vi "Set Position For Align Or Distribute.vi"(8 "Error In":errorcluster, 9 "Position":i32, 10 "Vertical? (F: Horizontal)":bool, 11 "Splitter in":refnum<class "Splitter.lvclass">) -> (0 "Error Out":errorcluster, 3 "Splitter out":refnum<class "Splitter.lvclass">)   [LabVIEW 2017, in "Splitter.lvclass"]
uses:
  Splitter.lvclass
  Splitter.lvclass/Splitter.ctl
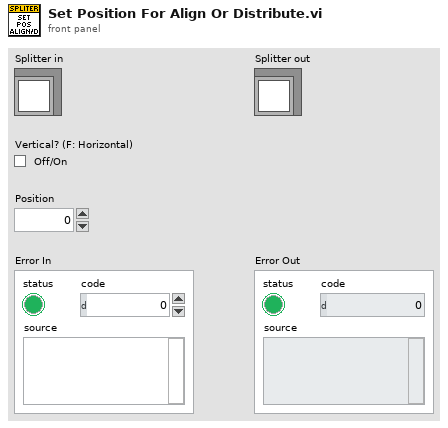
[diagram p1: front panel]
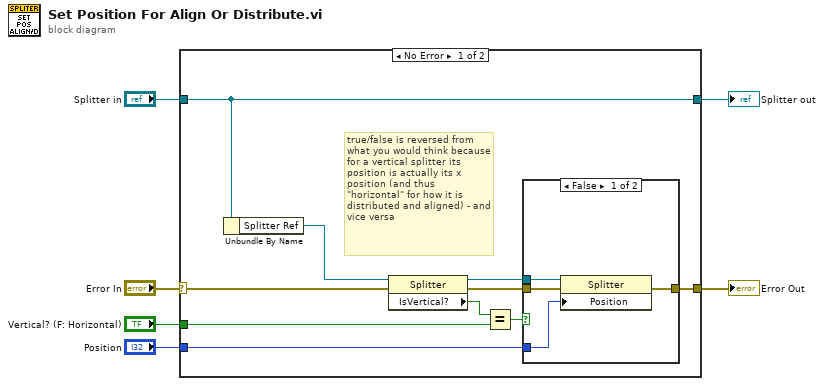
[diagram p0: block diagram]
diagram:
  n1 = case shown="No Error" "Error In" {
    selector: "Error In" -> [w15 w22]
    tunnel: "Splitter in" -> [w12 w23]
    tunnel: [w8 w22] -> w4
    tunnel: "Vertical? (F: Horizontal)" -> [w13 _]
    tunnel: [w12 w23] -> w2
    tunnel: "Position" -> [w7 _]
    frame No Error {
      # "true/false is reversed from what you would think because for a vertical splitter its position is actually its x position (and thus \"horizontal\" for how it is distributed and aligned) - and vice versa"
      n2 = Unbundle By Name(w12) -> ("Splitter Ref"=w16:refnum<vi>)
      n3 = property class="Splitter"(reference=w16, error in=w15) -> (reference out=w9:refnum<vi>, error out=w11:errorcluster, "IsVertical?"=w14:bool)
      n4 = Equal?(x=w14, y=w13) -> (x = y?=w10:bool)
      n5 = case shown="False" w10 {
        tunnel: w11 -> [w20 w21]
        tunnel: w9 -> [w19 _]
        tunnel: [w18 w21] -> w8
        tunnel: w7 -> [w17 _]
        frame False {
          n6 = property class="Splitter"(reference=w19, error in=w20, "Position"=w17) -> (error out=w18:errorcluster)  [unwired: 1 out]
        }
        frame True {
        }
      }
    }
    frame Error {
    }
  }
  "Splitter out" <- w2
  "Error Out" <- w4
